vi "part a.vi"() -> ()   [LabVIEW 2020]
uses:
  tree--cluster.ctl
panel:
  out "sum":i16
  out "Map":T1[][](array[typedef])
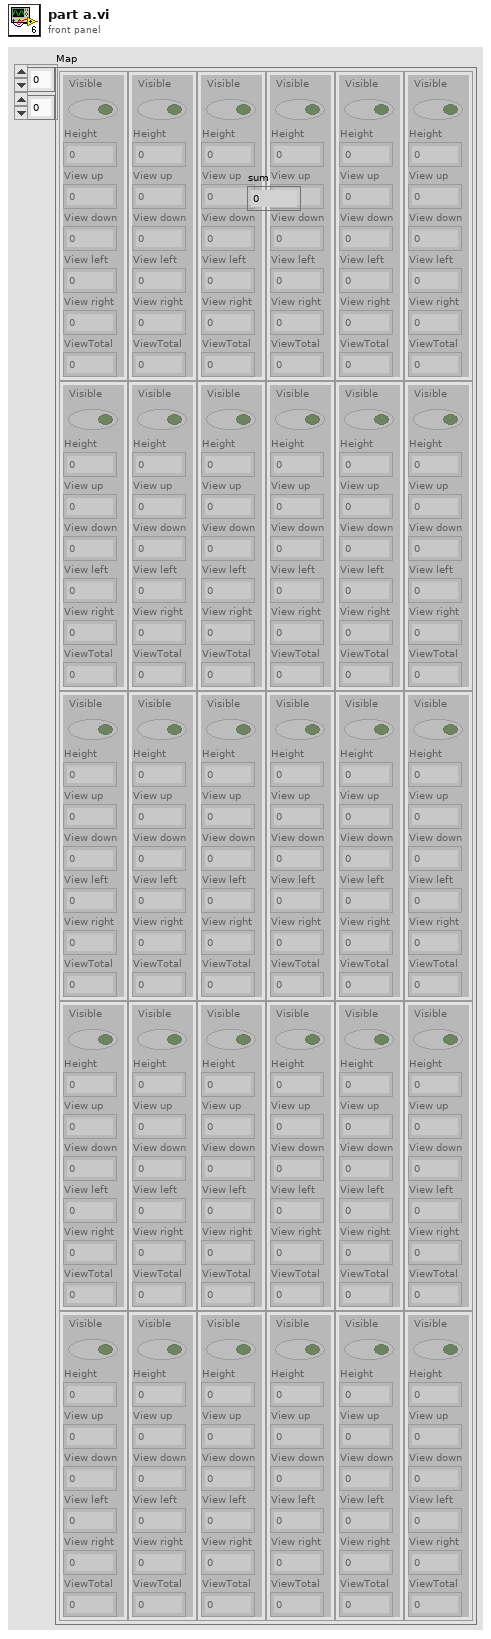
[diagram p1: front panel]
types:
  T1 = typedef "tree--cluster.ctl" = cluster{"Visible":bool, "Height":i32, "View up":i32, "View down":i32, "View left":i32, "View right":i32, "ViewTotal":i32}
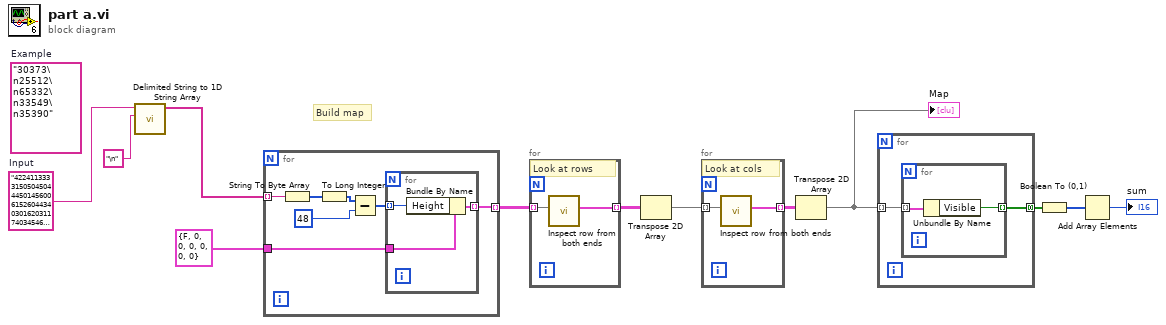
[diagram p0: block diagram]
diagram:
  w1 = "422411333315050450444501456006152604434030162031174034546313212413064150120521030152355534203000121\n301324204451515335252342253126503010214314026675523135330307170405066545120014006214521335013332134\n410011302103513543254453460342420630261341511764171765703774273674310415535166643155002215230224343\n103430412453541534313620414103230457371320115213510406561165762764547335046351220043205123531400041\n431144033221543442550410360065613506340166441027415155772664554705330520251311025141223233351402243\n213325510034542655030015455216430162202777001070241326522045362063054665216550230550303504355415521\n..."  # Input
  (unwired) "30373\n25512\n65332\n33549\n35390"  # Example
  # "Build map"
  n1 = call <vilib>:"Delimited String to 1D String Array.vi"("delimiter"="\n", "delimited string"=w1) -> ("string array"=w3:string[])  [unwired: 9 in]
  n2 = for {
    tunnel: w3 -> [w19] mode=indexing
    tunnel: [w13] -> w12 mode=indexing
    tunnel: T1 {"Visible"=FALSE, "Height"=0, "View up"=0, "View down"=0, "View left"=0, "View right"=0, "ViewTotal"=0} ("Tree") -> [w14]
    n3 = String To Byte Array(string=w19) -> (unsigned byte array=w18:u8[])
    n4 = To Long Integer(number=w18) -> (32bit integer=w16:i32[])
    n5 = Subtract(x=w16, y=48) -> (x-y=w15:i32[])
    n6 = for {
      tunnel: w15 -> [w21] mode=indexing
      tunnel: w14 -> [w22]
      tunnel: [w20] -> w13 mode=indexing
      n7 = Bundle By Name(cluster=w22, "Height"=w21) -> (w20:T1)
    }
  }
  n8 = for {
    tunnel: w12 -> [w24] mode=indexing
    tunnel: [w23] -> w9 mode=indexing
    # "Look at rows"
    n9 = call "Inspect row from both ends.vi"("Trees in"=w24) -> ("Trees out"=w23:T1[])  [unwired: 10 in]
  }
  n10 = Transpose 2D Array(2D array=w9) -> (transposed array=w11:T1[][])
  n11 = for {
    tunnel: w11 -> [w26] mode=indexing
    tunnel: [w25] -> w10 mode=indexing
    # "Look at cols"
    n12 = call "Inspect row from both ends.vi"("Trees in"=w26) -> ("Trees out"=w25:T1[])  [unwired: 10 in]
  }
  n13 = Transpose 2D Array(2D array=w10) -> (transposed array=w8:T1[][])
  "Map" <- w8
  n14 = for {
    tunnel: w8 -> [w28] mode=indexing
    tunnel: [w27] -> w7 mode=concatenating
    n15 = for {
      tunnel: w28 -> [w30] mode=indexing
      tunnel: [w29] -> w27 mode=indexing
      n16 = Unbundle By Name(w30) -> ("Visible"=w29:bool)
    }
  }
  n17 = Boolean To (0,1)(Boolean=w7) -> (0, 1=w6:i16[])
  n18 = Add Array Elements(numeric array=w6) -> (sum=→"sum":i16)
